vi "Adjust Absolute Offsets.vi"(9 "Top In":i32, 10 "Left In":i32, 11 "Coordinates in":T1) -> (1 "Top Out":i32, 2 "Left Out":i32, 3 "Coordinates out":T1)   [LabVIEW 2017, in "Front Panel Publisher.lvlib" / "Web Front Panel.lvclass"]
doc: "This VI will adjust the coorinates by a constant inside, which correspond to the HTML border used."
uses:
  Web Front Panel.lvclass
  Front Panel Objects/Object_class/Coordinates.ctl
  Front Panel Objects/Object_class/Object.lvclass
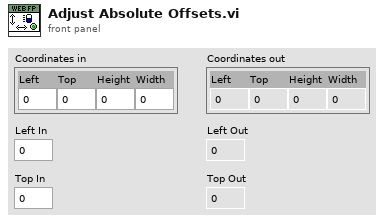
[diagram p1: front panel]
types:
  T1 = typedef "Front Panel Publisher.lvlib/Object.lvclass/Coordinates.ctl" = cluster{"Left":i32, "Top":i32, "Height":u32, "Width":u32}
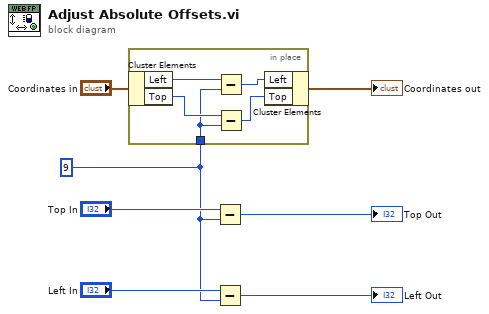
[diagram p0: block diagram]
diagram:
  w3 = 9 ("y")
  n1 = in-place {
    in-place-border: w3 -> [w8]
    n2 = in-place-cluster #1("Coordinates in") -> ("Left"=w12:i32, "Top"=w11:i32)
    n3 = Subtract(x=w12, y=w8) -> (x-y=w10:i32)
    n4 = Subtract(x=w11, y=w8) -> (x-y=w9:i32)
    n5 = in-place-cluster #1("Left"=w10, "Top"=w9) -> (→"Coordinates out":T1)
  }
  n6 = Subtract(x="Top In", y=w3) -> (x-y=→"Top Out":i32)
  n7 = Subtract(x="Left In", y=w3) -> (x-y=→"Left Out":i32)
